vi "MCA_ReadConfig.vi"() -> (0 "数据刷新频率":u16, 1 "测量最多花费的时间（秒）：":u16=1800, 2 "甄别后阈值":u16=100, 3 "甄别前阈值":u16=200, 4 "寻峰灵敏度":u16=8, 5 "最大道数":u16=1024, 6 "数据文件路径":path, 7 "信号极性":bool=TRUE, 11 "是否滤波":bool)   [LabVIEW 2014]
uses:
  <vilib>/Utility/config.llb/Read Key (U32).vi
  <vilib>/Utility/config.llb/Read Key (Path).vi
  <vilib>/Utility/config.llb/Read Key (Boolean).vi
  <vilib>/Utility/config.llb/NI_LVConfig.lvlib
panel:
  out "file or folder exists?":bool caption="文件或文件夹存在？"
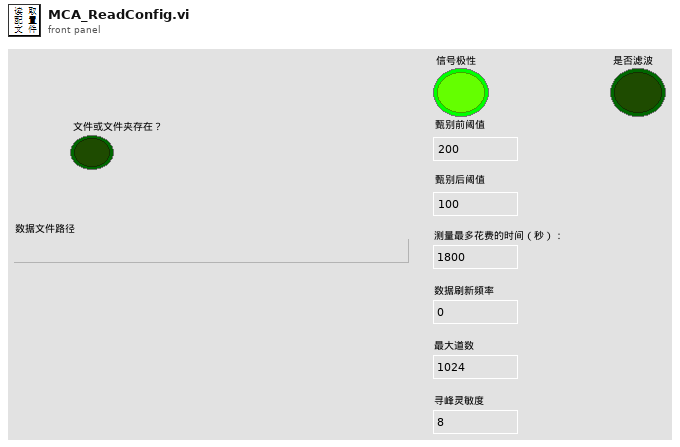
[diagram p1: front panel]
types:
  T1 = typedef "NI_LVConfig.lvlib/Config Data RefNum.ctl" = refnum<k1>
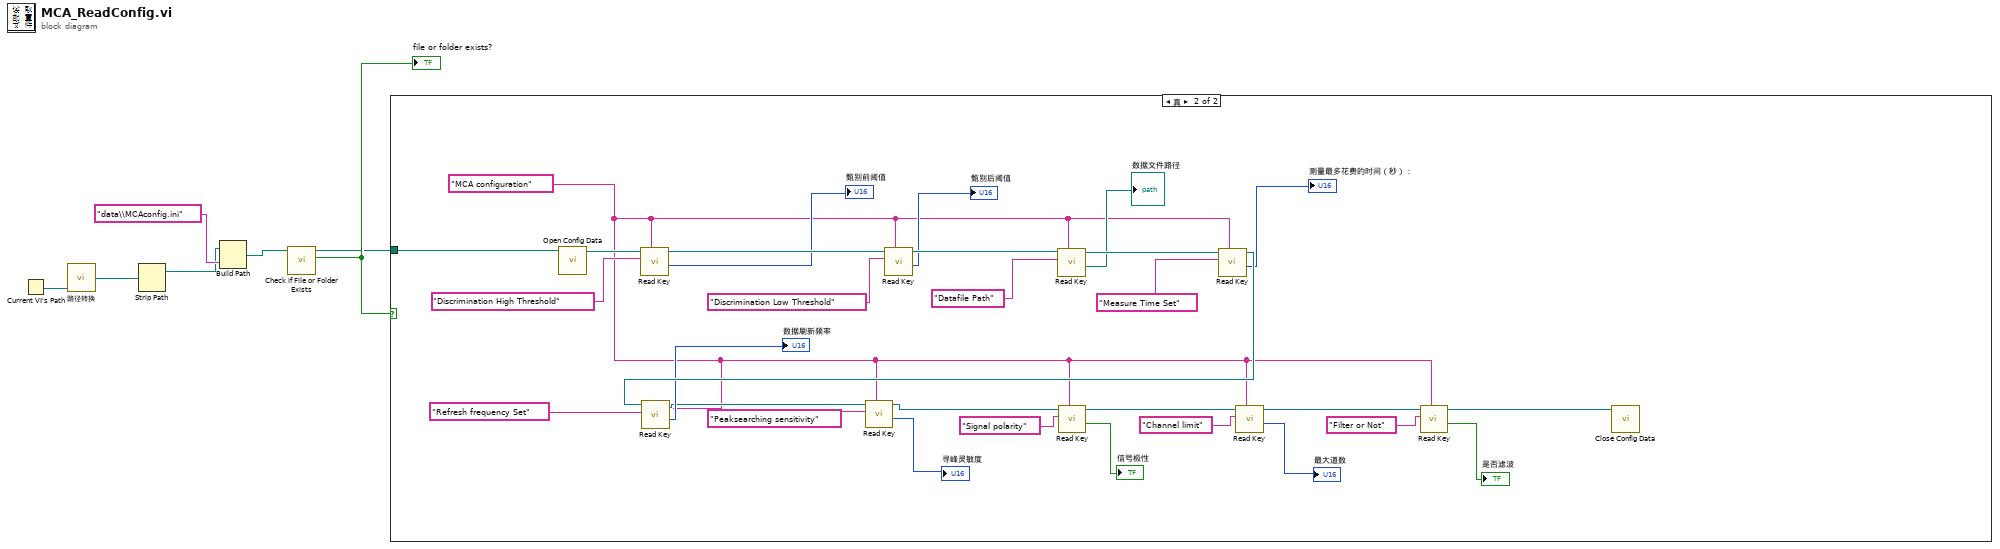
[diagram p0: block diagram]
diagram:
  n1 = Current VI's Path() -> (path=w1:path)
  n2 = call "路径转换.vi"("input path"=w1) -> ("output path"=w2:path)
  n3 = Strip Path(path=w2) -> (stripped path=w3:path)  [unwired: 1 out]
  n4 = Build Path(base path=w3, name or relative path="data\\MCAconfig.ini" ("名称或相对路径")) -> (appended path=w5:path)
  n5 = call <vilib>:"Check if File or Folder Exists.vi"("path"=w5) -> ("file or folder exists?"=w7:bool, "dup path"=w6:path)  [unwired: 8 in, 1 out]
  "file or folder exists?" <- w7
  n6 = case shown="真" w7 {
    tunnel: w6 -> [_ w22]
    frame False {
    }
    frame True {
      w11 = "MCA configuration" ("section")
      n7 = call <vilib>:"Open Config Data.vi"("configuration file path"=w22) -> ("refnum"=w37:T1)  [unwired: 8 in, 2 out]
      n8 = call-poly <vilib>:"Read Key.vi"("section"=w11, "key"="Discrimination High Threshold", "refnum"=w37) -> ("value"=→"甄别前阈值":u32, "refnum out"=w35:T1)  [unwired: 5 in, 2 out]
      n9 = call-poly <vilib>:"Read Key.vi"("section"=w11, "key"="Discrimination Low Threshold", "refnum"=w35) -> ("value"=→"甄别后阈值":u32, "refnum out"=w32:T1)  [unwired: 5 in, 2 out]
      n10 = call-poly <vilib>:"Read Key.vi"("section"=w11, "key"="Datafile Path", "refnum"=w32) -> ("value"=→"数据文件路径":path, "refnum out"=w31:T1)  [unwired: 5 in, 2 out]
      n11 = call-poly <vilib>:"Read Key.vi"("section"=w11, "key"="Measure Time Set", "refnum"=w31) -> ("value"=→"测量最多花费的时间（秒）：":u32, "refnum out"=w29:T1)  [unwired: 5 in, 2 out]
      n12 = call-poly <vilib>:"Read Key.vi"("section"=w11, "key"="Refresh frequency Set", "refnum"=w29) -> ("value"=→"数据刷新频率":u32, "refnum out"=w21:T1)  [unwired: 5 in, 2 out]
      n13 = call-poly <vilib>:"Read Key.vi"("section"=w11, "key"="Peaksearching sensitivity", "refnum"=w21) -> ("value"=→"寻峰灵敏度":u32, "refnum out"=w18:T1)  [unwired: 5 in, 2 out]
      n14 = call-poly <vilib>:"Read Key.vi"("section"=w11, "key"="Signal polarity", "refnum"=w18) -> ("value"=→"信号极性":bool, "refnum out"=w16:T1)  [unwired: 5 in, 2 out]
      n15 = call-poly <vilib>:"Read Key.vi"("section"=w11, "key"="Channel limit", "refnum"=w16) -> ("value"=→"最大道数":u32, "refnum out"=w13:T1)  [unwired: 5 in, 2 out]
      n16 = call-poly <vilib>:"Read Key.vi"("section"=w11, "key"="Filter or Not", "refnum"=w13) -> ("value"=→"是否滤波":bool, "refnum out"=w8:T1)  [unwired: 5 in, 2 out]
      n17 = call <vilib>:"Close Config Data.vi"("refnum"=w8) -> ()  [unwired: 9 in, 2 out]
    }
  }
